vi "Calibration_Main.vi"() -> ()   [LabVIEW 2017]
uses:
  <vilib>/userdefined/High Color/IMAQdx.ctl
panel:
  in  "Tab Control":T1(tab)
  out "Shot Success":bool
  in  "Kick":bool
  in  "stop":bool
  out "error out":errorcluster
  out "ImageOut":T2(plugin-control)
  in  "Session In":T3
  out "Horizontal Edges":T4(array[cluster]) {"Point2 (Real-World)"."Y" format="%.2f"; "Point2 (Real-World)"."X" format="%.2f"; "Point1 (Real-World)"."Y" format="%.2f"; "Point1 (Real-World)"."X" format="%.2f"; "Point2 (Pixels)"."Y" format="%.2f"; "Point2 (Pixels)"."X" format="%.2f"; "Point1 (Pixels)"."Y" format="%.2f"; "Point1 (Pixels)"."X" format="%.2f"}
  out "Vertical Edges":T4(array[cluster]) {"Point2 (Real-World)"."Y" format="%.2f"; "Point2 (Real-World)"."X" format="%.2f"; "Point1 (Real-World)"."Y" format="%.2f"; "Point1 (Real-World)"."X" format="%.2f"; "Point2 (Pixels)"."Y" format="%.2f"; "Point2 (Pixels)"."X" format="%.2f"; "Point1 (Pixels)"."Y" format="%.2f"; "Point1 (Pixels)"."X" format="%.2f"}
  out "error out 2":errorcluster
  out "Players":T5(array[cluster]) {"Position"."Y" format="%.2f"; "Position"."X" format="%.2f"}
  out "ChosenAngle":dbl
  out "ChosenPathIdx":i32
  out "ChosenEnergy":dbl
  out "Kicker XY":cluster{dbl, dbl}
  out "Puck":T5(array[cluster]) {"Position"."Y" format="%.2f"; "Position"."X" format="%.2f"}
  out "Image Out":T2(plugin-control)
  out "Histogram Graph":cluster{dbl[], dbl[]}(graph)
  in  "Brightness Input":i64(slide) scale=0.0..255.0
  in  "Contrast Input":dbl(slide) scale=0.0..1.0
  in  "Threshold Input":sgl(slide) scale=0.0..255.0
  in  "Stop":bool
  out "Camera Setup Error":errorcluster
  out "Threshold Image":T2(plugin-control)
  out "Before Image":T2(plugin-control)
  out "Histogram Statistics":T6
  out "Quality Check Variables":T7
  in  "Reference":bool
  in  "stop 2":bool
  out "Image 2":T2(plugin-control)
  in  "Calibrate":bool
  in  "Grid Descriptor":cluster{"X Step":sgl, "Y Step":sgl, "Unit":T8}={"X Step"=5.0, "Y Step"=5.0, "Unit"=enum."Millimeter"}
  in  "File Path":path
  out "Calibration Error":errorcluster
  out "Corrected Image":T2(plugin-control)
  out "Y":sgl
  out "X":sgl
  out "X 2":sgl
  out "Y 2":sgl
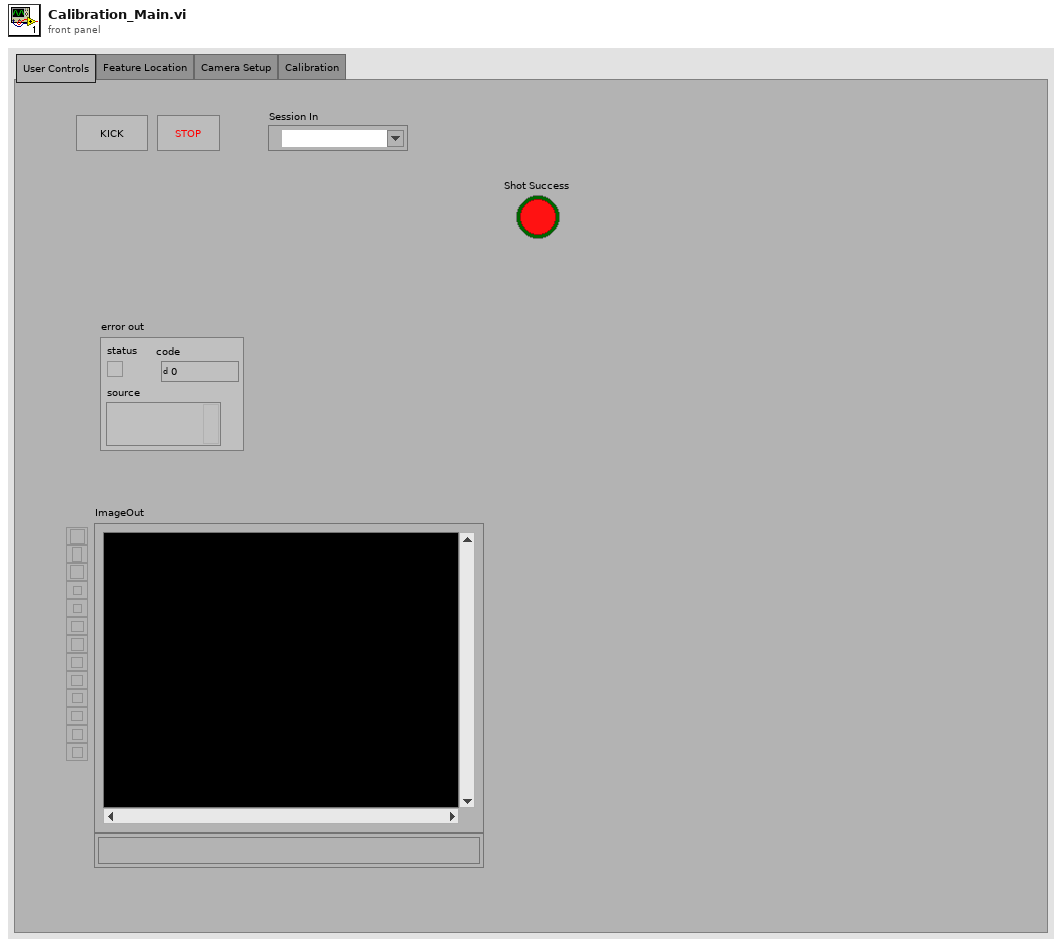
[diagram p1: front panel]
types:
  T1 = enum32{"User Controls", "Feature Location", "Camera Setup", "Calibration"}
  T2 = typedef "IMAQ Image.ctl" = refnum<image>
  T3 = typedef "IMAQdx.ctl" = refnum<k21>
  T4 = cluster{"Point1 (Pixels)":cluster{"X":sgl, "Y":sgl}, "Point2 (Pixels)":cluster{"X":sgl, "Y":sgl}, "Point1 (Real-World)":cluster{"X":sgl, "Y":sgl}, "Point2 (Real-World)":cluster{"X":sgl, "Y":sgl}, "Angle (Pixel)":dbl, "Angle (Real-World)":dbl, "Score":dbl, "Straightness":dbl, "Average SNR (db)":dbl, "Calibration Valid":bool}[]
  T5 = cluster{"Position":cluster{"X":sgl, "Y":sgl}, "Radius":dbl, "Score":dbl}[]
  T6 = cluster{"Mean Value":sgl, "Standard  Variation":sgl, "Range":sgl}
  T7 = cluster{"Mean +":dbl, "Mean -":dbl, "Within Range":bool}
  T8 = typedef "Image Unit" = enum32{"Undefined", "Angström", "Micrometer", "Millimeter", "Centimeter", "Meter", "Kilometer", "Microinch", "Inch", "Feet", "Nautical miles", "Standard miles", "Steps"}
  T9 = cluster{"Brightness":i64, "Contrast":dbl, "Threshold":sgl}
  T10 = typedef "IMAQ Coordinate System" = cluster{"Reference System":cluster{"Origin":cluster{"X":sgl, "Y":sgl}, "Angle (deg)":sgl, "Axis Reference":u32}, "Measurement System":cluster{"Origin":cluster{"X":sgl, "Y":sgl}, "Angle (deg)":sgl, "Axis Reference":u32}}
  T11 = cluster{"Circles[0]":cluster{"Position":cluster{"X":sgl, "Y":sgl}, "Radius":dbl, "Score":dbl}, "Circles[1]":cluster{"Position":cluster{"X":sgl, "Y":sgl}, "Radius":dbl, "Score":dbl}, "Circles[2]":cluster{"Position":cluster{"X":sgl, "Y":sgl}, "Radius":dbl, "Score":dbl}, "Circles[3]":cluster{"Position":cluster{"X":sgl, "Y":sgl}, "Radius":dbl, "Score":dbl}, "Circles[4]":cluster{"Position":cluster{"X":sgl, "Y":sgl}, "Radius":dbl, "Score":dbl}, "Circles[5]":cluster{"Position":cluster{"X":sgl, "Y":sgl}, "Radius":dbl, "Score":dbl}, "Circles[6]":cluster{"Position":cluster{"X":sgl, "Y":sgl}, "Radius":dbl, "Score":dbl}, "Circles[7]":cluster{"Position":cluster{"X":sgl, "Y":sgl}, "Radius":dbl, "Score":dbl}, "Circles[8]":cluster{"Position":cluster{"X":sgl, "Y":sgl}, "Radius":dbl, "Score":dbl}}
  T12 = cluster{"Ptwx":dbl[], "Ptwy":dbl[], "Ptfx":dbl[], "Ptfy":dbl[], "DorR":i32[]}
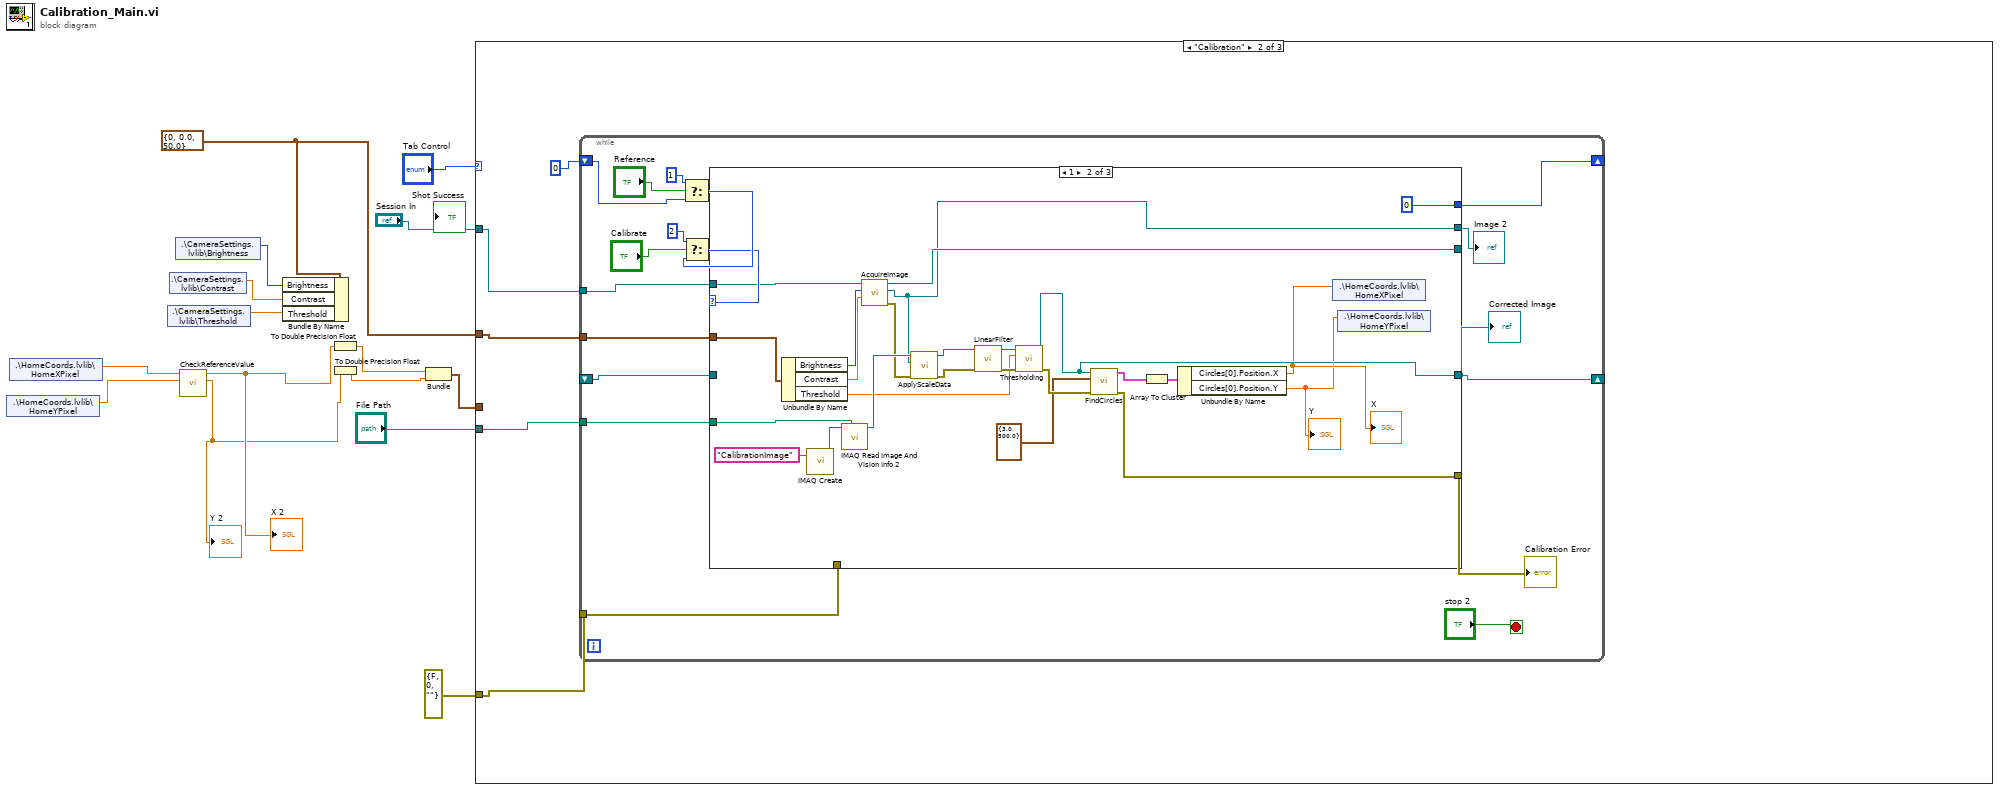
[diagram p0: block diagram]
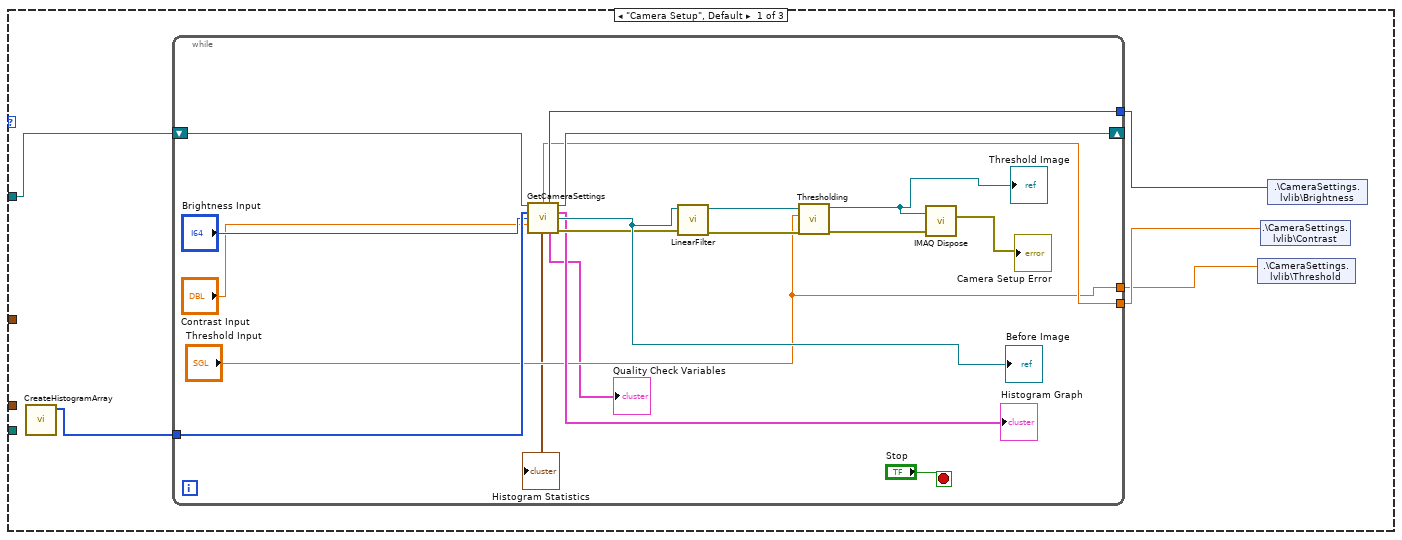
[diagram p2: hidden frame]
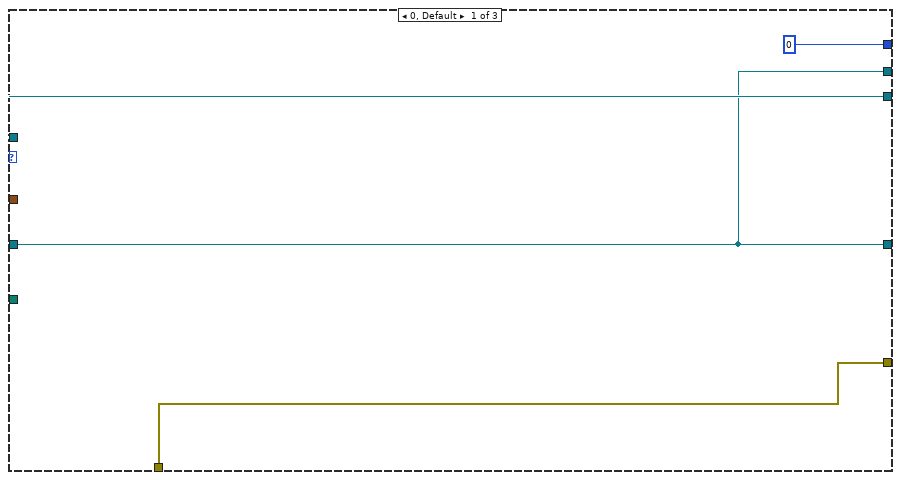
[diagram p3: hidden frame]
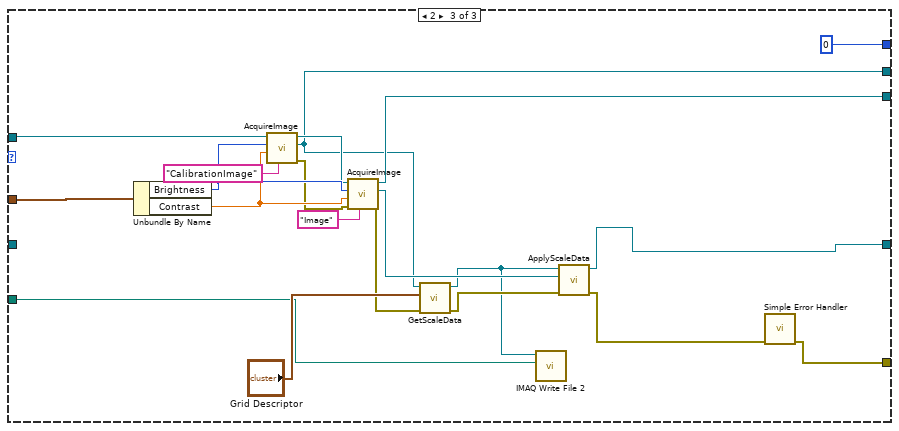
[diagram p4: hidden frame]
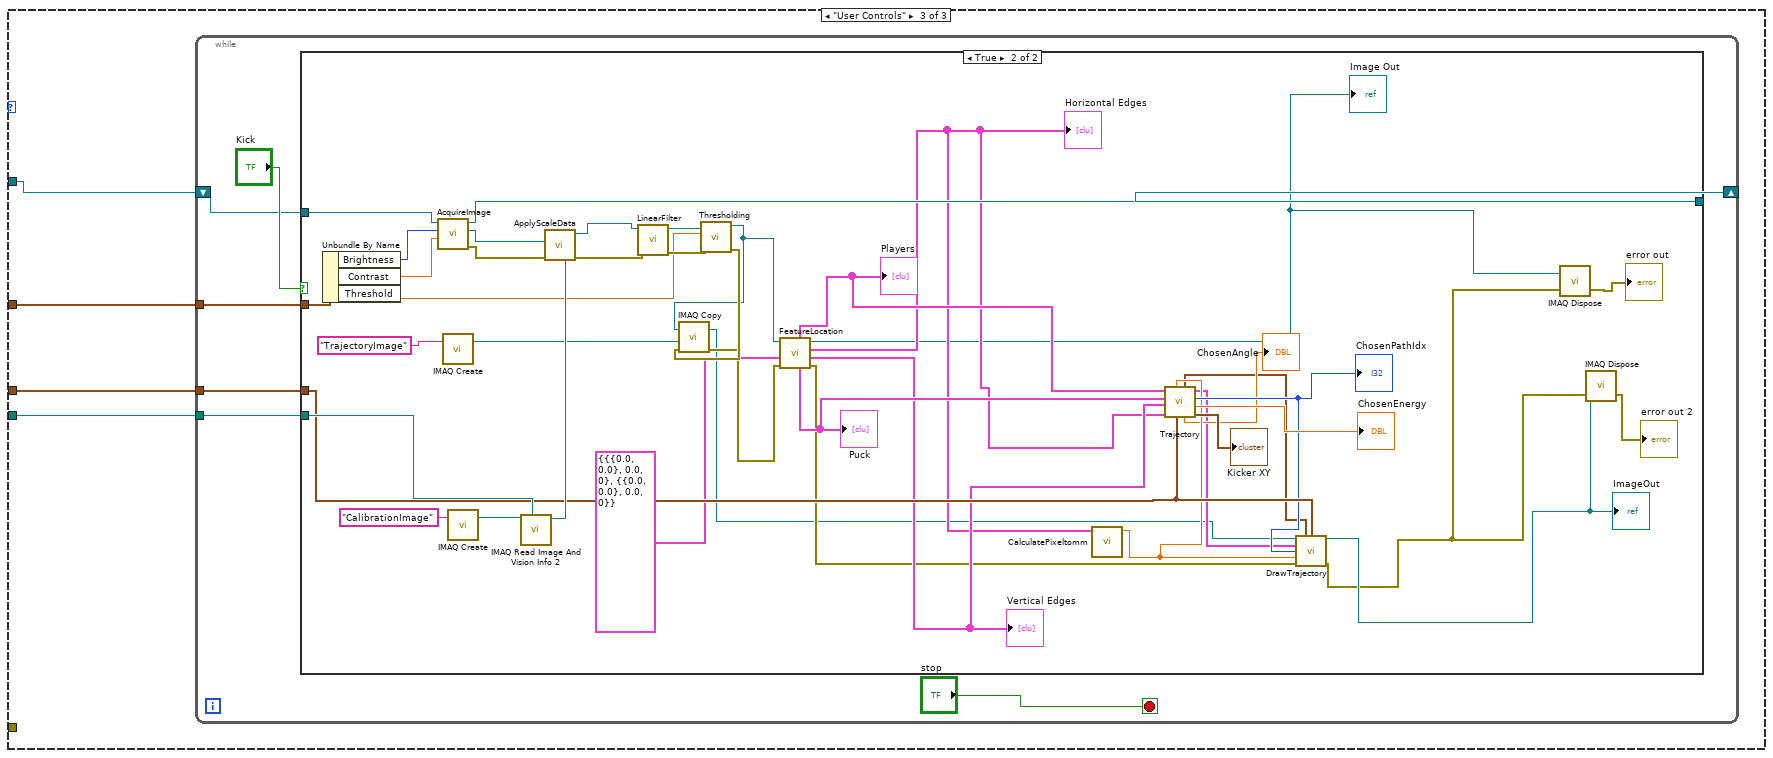
[diagram p5: hidden frame]
diagram:
  w9 = T9 {"Brightness"=0, "Contrast"=0.0, "Threshold"=50.0} ("CameraSettings")
  n1 = shared-variable ".\\HomeCoords.lvlib\\HomeYPixel"() -> (w3:sgl)  [unwired: 1 in, 1 out]
  n2 = shared-variable ".\\HomeCoords.lvlib\\HomeXPixel"() -> (w4:sgl)  [unwired: 1 in, 1 out]
  n3 = shared-variable ".\\CameraSettings.lvlib\\Threshold"() -> (w7:sgl)  [unwired: 1 in, 1 out]
  n4 = shared-variable ".\\CameraSettings.lvlib\\Contrast"() -> (w8:dbl)  [unwired: 1 in, 1 out]
  n5 = shared-variable ".\\CameraSettings.lvlib\\Brightness"() -> (w10:i64)  [unwired: 1 in, 1 out]
  n6 = call "CheckReferenceValue.vi"("YCoordIn"=w3, "XCoordIn"=w4) -> ("YCoordOut"=w1:sgl, "XCoordOut"=w2:sgl)  [unwired: 8 in]
  "X 2" <- w2
  "Y 2" <- w1
  n7 = Bundle By Name(cluster=w9, "Brightness"=w10, "Contrast"=w8, "Threshold"=w7) -> ()  [unwired: 1 out]
  n8 = To Double Precision Float(number=w2) -> (double precision float=w6:dbl)
  n9 = To Double Precision Float(number=w1) -> (double precision float=w5:dbl)
  n10 = Bundle(w6, w5) -> (w11:cluster{dbl, dbl})  [unwired: 1 in]
  n11 = case shown="\"Calibration\"" "Tab Control" {
    tunnel: "Session In" -> [w19 w44 w114]
    tunnel: w9 -> [_ w43 w112]
    tunnel: "File Path" -> [_ w42 w113]
    tunnel: errorcluster {"status"=FALSE, "code"=0, "source"=""} ("error out") -> [_ w40 _]
    tunnel: w11 -> [_ _ w111]
    frame "Camera Setup", Default {
      n12 = call "CreateHistogramArray.vi"() -> ("Array"=w20:i32[])  [unwired: 11 in]
      n13 = while {
        shift-right: [w29] -> _
        shift-left: w19 -> [w37]
        tunnel: w20 -> [w36]
        tunnel: [w24] -> w17
        tunnel: ["Threshold Input"] -> w16
        tunnel: [w25] -> w18
        stop <- "Stop" stop-if-true
        n14 = call "GetCameraSettings.vi"("Session In"=w37, "Array"=w36, "Brightness"="Brightness Input", "Contrast"="Contrast Input") -> ("Contrast"=w24:dbl, "Brightness"=w25:i64, "Session Out"=w29:T3, "Histogram Graph"=→"Histogram Graph":cluster{dbl[], dbl[]}, "Image"=w28:T2, "Histogram Statistics"=→"Histogram Statistics":T6, "Quality Check Variables"=→"Quality Check Variables":T7, "error out"=w27:errorcluster)  [unwired: 4 in]
        "Before Image" <- w28
        n15 = call "LinearFilter.vi"("error in (no error)"=w27, "Image Src"=w28) -> ("error out"=w32:errorcluster, "Image"=w33:T2)  [unwired: 8 in]
        n16 = call "Thresholding.vi"("error in (no error)"=w32, "Threshold Value"="Threshold Input", "Image Src"=w33) -> ("error out"=w31:errorcluster, "Image"=w30:T2)  [unwired: 7 in]
        "Threshold Image" <- w30
        n17 = call "IMAQ Dispose"("Image"=w30, "error in (no error)"=w31) -> ("error out"=→"Camera Setup Error":errorcluster)  [unwired: 4 in]
      }
      n18 = shared-variable ".\\CameraSettings.lvlib\\Threshold"(w16) -> ()  [unwired: 1 in, 1 out]
      n19 = shared-variable ".\\CameraSettings.lvlib\\Contrast"(w17) -> ()  [unwired: 1 in, 1 out]
      n20 = shared-variable ".\\CameraSettings.lvlib\\Brightness"(w18) -> ()  [unwired: 1 in, 1 out]
    }
    frame "Calibration" {
      n21 = while {
        tunnel: w44 -> [w61]
        tunnel: w43 -> [w60]
        tunnel: w42 -> [w58]
        shift-right: [w57] -> _
        shift-left: 0 -> [w51]
        shift-right: [w45] -> _
        shift-left: _ -> [w48]
        tunnel: w40 -> [w49]
        stop <- "stop 2" stop-if-true
        n22 = Select(t=1, s="Reference", f=w51) -> (s? t:f=w54:i32)
        n23 = Select(t=2, s="Calibrate", f=w54) -> (s? t:f=w50:i32)
        n24 = case shown="1" w50 {
          tunnel: w61 -> [w65 w88 w110]
          tunnel: w60 -> [_ w86 w109]
          tunnel: [w65 w87 w102] -> _
          tunnel: w58 -> [_ w84 w93]
          tunnel: [w63 w69 w104] -> w47
          tunnel: [w62 w70 w94] -> w45
          tunnel: [0 0 0] -> w57
          tunnel: w49 -> [w63 _ _]
          tunnel: w48 -> [w62 _ _]
          tunnel: [w62 w80 w91] -> w46
          frame 0, Default {
          }
          frame 1 {
            n25 = Unbundle By Name(w86) -> ("Brightness"=w90:i64, "Contrast"=w89:dbl, "Threshold"=w74:sgl)
            n26 = call "IMAQ Create"("Image Name"="CalibrationImage") -> ("New Image"=w82:T2)  [unwired: 4 in, 1 out]
            n27 = call "IMAQ Read Image And Vision Info 2"("File Path"=w84, "Image"=w82) -> ("Image Out"=w81:T2)  [unwired: 7 in, 2 out]
            n28 = call "AcquireImage.vi"("Contrast"=w89, "Brightness"=w90, "Session In"=w88) -> ("error out"=w77:errorcluster, "Image"=w80:T2, "Session Out"=w87:T3)  [unwired: 5 in]
            n29 = call "ApplyScaleData.vi"("error in (no error)"=w77, "ImageIn"=w80, "CalibImage"=w81) -> ("error out"=w76:errorcluster, "Corrected Image"=w79:T2)  [unwired: 7 in]
            n30 = call "LinearFilter.vi"("error in (no error)"=w76, "Image Src"=w79) -> ("error out"=w75:errorcluster, "Image"=w78:T2)  [unwired: 8 in]
            n31 = call "Thresholding.vi"("error in (no error)"=w75, "Threshold Value"=w74, "Image Src"=w78) -> ("error out"=w73:errorcluster, "Image"=w70:T2)  [unwired: 7 in]
            n32 = call "FindCircles.vi"("error in (no error)"=w73, "Circle Descriptor"=cluster{"Min Radius":dbl, "Max Radius":dbl} {"Min Radius"=3.0, "Max Radius"=500.0}, "Image"=w70) -> ("error out"=w69:errorcluster, "Circles"=w72:T5)  [unwired: 6 in, 1 out]
            n33 = Array To Cluster(array=w72) -> (cluster=w71:T11)
            n34 = Unbundle By Name(w71) -> ("Circles[0].Position.X"=w68:sgl, "Circles[0].Position.Y"=w67:sgl)
            "X" <- w68
            "Y" <- w67
            n35 = shared-variable ".\\HomeCoords.lvlib\\HomeXPixel"(w68) -> ()  [unwired: 1 in, 1 out]
            n36 = shared-variable ".\\HomeCoords.lvlib\\HomeYPixel"(w67) -> ()  [unwired: 1 in, 1 out]
          }
          frame 2 {
            n37 = Unbundle By Name(w109) -> ("Brightness"=w107:i64, "Contrast"=w106:dbl)
            n38 = call "AcquireImage.vi"("Image Name"="CalibrationImage", "Contrast"=w106, "Brightness"=w107, "Session In"=w110) -> ("error out"=w105:errorcluster, "Image"=w91:T2, "Session Out"=w103:T3)  [unwired: 4 in]
            n39 = call "AcquireImage.vi"("Image Name"="Image", "error in"=w105, "Contrast"=w106, "Brightness"=w107, "Session In"=w103) -> ("error out"=w97:errorcluster, "Image"=w98:T2, "Session Out"=w102:T3)  [unwired: 3 in]
            n40 = call "GetScaleData.vi"("error in (no error)"=w97, "Grid Descriptor"="Grid Descriptor", "Image Src"=w91) -> ("error out"=w96:errorcluster, "Image"=w92:T2)  [unwired: 7 in]
            n41 = call-poly "IMAQ Write File 2"("File Path"=w93, "Image"=w92) -> ()  [unwired: 8 in, 2 out]
            n42 = call "ApplyScaleData.vi"("error in (no error)"=w96, "ImageIn"=w98, "CalibImage"=w92) -> ("error out"=w95:errorcluster, "Corrected Image"=w94:T2)  [unwired: 7 in]
            n43 = call <vilib>:"Simple Error Handler.vi"("error in (no error)"=w95) -> ("error out"=w104:errorcluster)  [unwired: 4 in, 4 out]
          }
        }
        "Calibration Error" <- w47
        "Image 2" <- w46
        "Corrected Image" <- w45
      }
    }
    frame "User Controls" {
      n44 = while {
        shift-right: [w119] -> _
        shift-left: w114 -> [w120]
        tunnel: w113 -> [w117]
        tunnel: w112 -> [w116]
        tunnel: w111 -> [w115]
        stop <- "stop" stop-if-true
        n45 = case shown="True" "Kick" {
          tunnel: w120 -> [w122 w150]
          tunnel: [w122 w160] -> w119
          tunnel: w117 -> [_ w163]
          tunnel: w116 -> [_ w158]
          tunnel: w115 -> [_ w152]
          frame False {
          }
          frame True {
            n46 = Unbundle By Name(w158) -> ("Brightness"=w149:i64, "Contrast"=w148:dbl, "Threshold"=w154:sgl)
            n47 = call "AcquireImage.vi"("Contrast"=w148, "Brightness"=w149, "Session In"=w150) -> ("error out"=w151:errorcluster, "Image"=w147:T2, "Session Out"=w160:T3)  [unwired: 5 in]
            n48 = call "IMAQ Create"("Image Name"="TrajectoryImage") -> ("New Image"=w144:T2)  [unwired: 4 in, 1 out]
            n49 = call "IMAQ Create"("Image Name"="CalibrationImage") -> ("New Image"=w161:T2)  [unwired: 4 in, 1 out]
            n50 = call "IMAQ Read Image And Vision Info 2"("File Path"=w163, "Image"=w161) -> ("Image Out"=w159:T2)  [unwired: 7 in, 2 out]
            n51 = call "ApplyScaleData.vi"("error in (no error)"=w151, "ImageIn"=w147, "CalibImage"=w159) -> ("error out"=w156:errorcluster, "Corrected Image"=w153:T2)  [unwired: 7 in]
            n52 = call "LinearFilter.vi"("error in (no error)"=w156, "Image Src"=w153) -> ("error out"=w155:errorcluster, "Image"=w157:T2)  [unwired: 8 in]
            n53 = call "Thresholding.vi"("error in (no error)"=w155, "Threshold Value"=w154, "Image Src"=w157) -> ("error out"=w141:errorcluster, "Image"=w126:T2)  [unwired: 7 in]
            n54 = call "IMAQ Copy"("error in (no error)"=w141, "Image Dst"=w144, "Image Src"=w126) -> ("error out"=w140:errorcluster, "Image Dst Out"=w124:T2)  [unwired: 3 in]
            n55 = call "FeatureLocation.vi"("error in (no error)"=w140, "Coordinate System"=T10 {"Reference System"={"Origin"={"X"=0.0, "Y"=0.0}, "Angle (deg)"=0.0, "Axis Reference"=0}, "Measurement System"={"Origin"={"X"=0.0, "Y"=0.0}, "Angle (deg)"=0.0, "Axis Reference"=0}}, "Image"=w126) -> ("error out"=w128:errorcluster, "Vertical Edges"=w136:T4, "Horizontal Edges"=w133:T4, "Image 2"=w125:T2, "Puck"=w137:T5, "Players"=w138:T5)  [unwired: 3 in]
            "Image Out" <- w125
            "Horizontal Edges" <- w133
            "Vertical Edges" <- w136
            "Players" <- w138
            "Puck" <- w137
            n56 = call "CalculatePixeltomm.vi"("Horizontal Edges"=w133) -> ("Pixel/mm"=w131:dbl)  [unwired: 10 in]
            n57 = call "Trajectory.vi"("HomeXY(pixels)"=w152, "PixelmmRatio"=w131, "Horizontal Edges"=w133, "Vertical Edges"=w136, "Puck"=w137, "Players"=w138) -> ("Kicker XY"=→"Kicker XY":cluster{dbl, dbl}, "ChosenEnergy"=→"ChosenEnergy":dbl, "ChosenPathIdx"=w132:i32, "TrajectoryArray"=w127:T12, "Angle"=→"ChosenAngle":dbl, "PuckCentre"=w129:cluster{"PuckX":sgl, "PuckY":sgl})
            "ChosenPathIdx" <- w132
            n58 = call "DrawTrajectory.vi"("Image"=w124, "PuckCentre"=w129, "HomePoint(pixels)"=w152, "TrajectoryArray"=w127, "ChosenPath"=w132, "Pixel/mm"=w131, "error in (no error)"=w128) -> ("ImageOut"=w142:T2, "error out"=w139:errorcluster)  [unwired: 7 in]
            "ImageOut" <- w142
            n59 = call "IMAQ Dispose"("Image"=w125, "error in (no error)"=w139) -> ("error out"=→"error out":errorcluster)  [unwired: 4 in]
            n60 = call "IMAQ Dispose"("Image"=w142, "error in (no error)"=w139) -> ("error out"=→"error out 2":errorcluster)  [unwired: 4 in]
          }
        }
      }
    }
  }
